vi "test_RemoteFgenSession_CallInitializeMeasurementLinkSessionWithAttachBehavior_RemoteSessionAttached.vi"(8 "error in":errorcluster) -> (0 "error out":errorcluster, 2 "result":string, 3 "pass":bool)   [LabVIEW 2020, in "MeasurementServerTests.lvlib"]
uses:
  MeasurementServerTests.lvlib
  Runtime/Sessions/niFGEN/Session Factory/Session Factory.lvclass
  Runtime/Sessions/Instrument/ISession Factory/Initialize and Close Session Behavior.ctl
  Runtime/Sessions/Instrument/ISession Factory/ISession Factory.lvclass
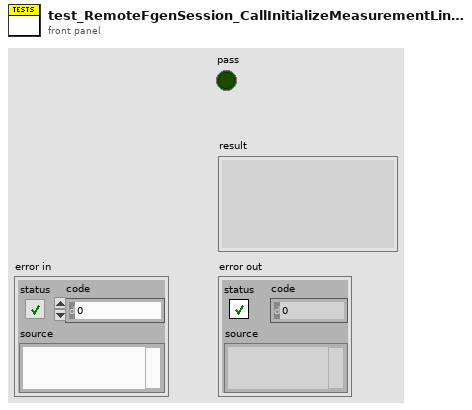
[diagram p1: front panel]
types:
  T1 = typedef "NI Session Management Instrument.lvlib/ISession Factory.lvclass/Remote Connection Options.ctl" = cluster{"session name":string, "address":string, "port":u32}
  T2 = typedef "NI Session Management Instrument.lvlib/ISession Factory.lvclass/Initialize and Close Session Behavior.ctl" = enum16{"Initialize and Close", "Attach and Detach", "Initialize and Detach", "Attach and Close"}
  T3 = typedef "NI Session Management Instrument.lvlib/ISession Factory.lvclass/Session Initialization Parameters.ctl" = cluster{"resource name":string, "session name":string}
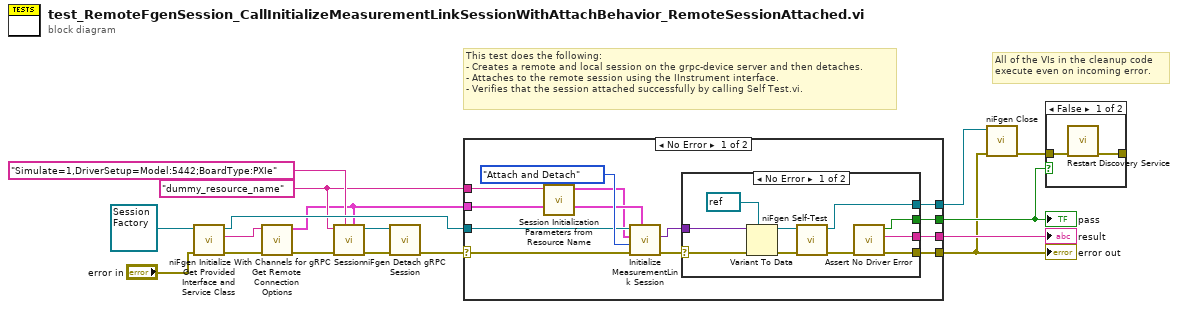
[diagram p0: block diagram]
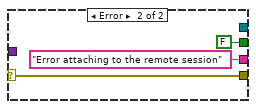
[diagram p2: hidden frame]
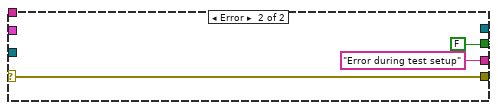
[diagram p3: hidden frame]
diagram:
  w4 = "dummy_resource_name" ("resource name")
  # "All of the VIs in the cleanup code\nexecute even on incoming error."
  # "This test does the following:\n- Creates a remote and local session on the grpc-device server and then detaches.\n- Attaches to the remote session using the IInstrument interface.\n- Verifies that the session attached successfully by calling Self Test.vi."
  n1 = call-dynamic "Get Provided Interface and Service Class.vi"("error in"="error in", "session factory in"=refnum<class "Session Factory.lvclass"> refnum ("MeasurementLink niFGEN.lvlib:Instrument.lvclass")) -> ("error out"=w13:errorcluster, "provided interface"=w12:string, "session factory out"=w10:refnum<class "Session Factory.lvclass">)  [unwired: 6 in, 1 out]
  n2 = call "Get Remote Connection Options.vi"("error in"=w13, "provided interface"=w12) -> ("error out"=w6:errorcluster, "remote connection options"=w3:T1)  [unwired: 8 in]
  n3 = call <instrlib>:"niFgen Initialize With Channels for gRPC Session.vi"("gRPC Options"=w3, "Option String"="Simulate=1,DriverSetup=Model:5442;BoardType:PXIe" ("option string"), "error in (no error)"=w6, "Resource Name"=w4) -> ("error out"=w7:errorcluster, "Instrument Handle Out"=w2:refnum<k15>)  [unwired: 6 in]
  n4 = call <instrlib>:"niFgen Detach gRPC Session.vi"("error in (no error)"=w7, "Instrument Handle"=w2) -> ("error out"=w8:errorcluster)  [unwired: 9 in]
  n5 = case shown="No Error" w8 {
    selector: w8 -> [w23 w43]
    tunnel: [w28 w43] -> w14
    tunnel: [w29 FALSE] -> w15
    tunnel: [w27 "Error during test setup" ("f")] -> w17
    tunnel: w10 -> [w22 _]
    tunnel: w3 -> [w21 _]
    tunnel: w4 -> [w20 _]
    tunnel: [w19 _] -> w1
    frame No Error {
      n6 = call "Session Initialization Parameters from Resource Name.vi"("resource name"=w20) -> ("session initialization parameters"=w18:T3)  [unwired: 10 in]
      n7 = call-dynamic "Initialize MeasurementLink Session.vi"("remote connection options"=w21, "error in"=w23, "initialize and close session behavior"=Initialize_and_Close_Session_Behavior."Attach and Detach", "session initialization parameters"=w18, "session factory in"=w22) -> ("error out"=w25:errorcluster, "session out"=w26:variant)  [unwired: 4 in, 1 out]
      n8 = case shown="No Error" w25 {
        selector: w25 -> [w38 w41]
        tunnel: [w32 FALSE] -> w29
        tunnel: [w30 w41] -> w28
        tunnel: [w31 "Error attaching to the remote session"] -> w27
        tunnel: w26 -> [w39 _]
        tunnel: [w33 _] -> w19
        frame No Error {
          n9 = Variant To Data(error in=w38, type=refnum<k15> refnum ("Instrument Handle Out"), Variant=w39) -> (data=w36:refnum<k15>, error out=w37:errorcluster)
          n10 = call <instrlib>:"niFgen Self-Test.vi"("error in (no error)"=w37, "Instrument Handle"=w36) -> ("error out"=w34:errorcluster, "Instrument Handle Out"=w33:refnum<k15>)  [unwired: 6 in, 2 out]
          n11 = call "Assert No Driver Error.vi"("error in"=w34) -> ("error out"=w30:errorcluster, "result"=w31:string, "pass?"=w32:bool)  [unwired: 8 in]
        }
        frame Error {
        }
      }
    }
    frame Error {
    }
  }
  "error out" <- w14
  "pass" <- w15
  "result" <- w17
  n12 = call <instrlib>:"niFgen Close.vi"("error in (no error)"=w14, "Instrument Handle"=w1) -> ("error out"=w16:errorcluster)  [unwired: 9 in]
  n13 = case shown="False" w15 {
    tunnel: w16 -> [w47 _]
    tunnel: [w46 _] -> _
    frame False {
      n14 = call "Restart Discovery Service.vi"("error in"=w47) -> ("error out"=w46:errorcluster)  [unwired: 10 in]
    }
    frame True {
    }
  }
